vi "eventlog.vi"(7 "httpRequestID":u32) -> ()   [LabVIEW 2011]
doc: "This VI is a state machine that can be ran from a Browser."
uses:
  server/database/Users/User Record.ctl
  <vilib>/wsapi/NI_WebServices.lvlib
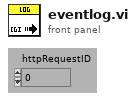
[diagram p1: front panel]
types:
  T1 = typedef "User Record.ctl" = cluster{"ixUser":i32, "sxUsername":string, "sLastName":string, "sFirstName":string, "sEmail":string, "sPassword":string, "tLoginTime":timestamp, "sLoginComputer":string, "fAdministrator":bool, "fRunSequences":bool, "fModifySequences":bool, "fRunScenarios":bool, "fModifyScenarios":bool, "fModifyTemplates":bool, "fModifyUsers":bool, "fModifyStations":bool, "fModifyFields":bool}
  T2 = typedef "Connection Refnum.ctl" = cluster{"Environment Handle":i32, "Connection Handle":i32}
  T3 = typedef "Keyed Array.ctl" = cluster{"keys":string[], "values":string[]}
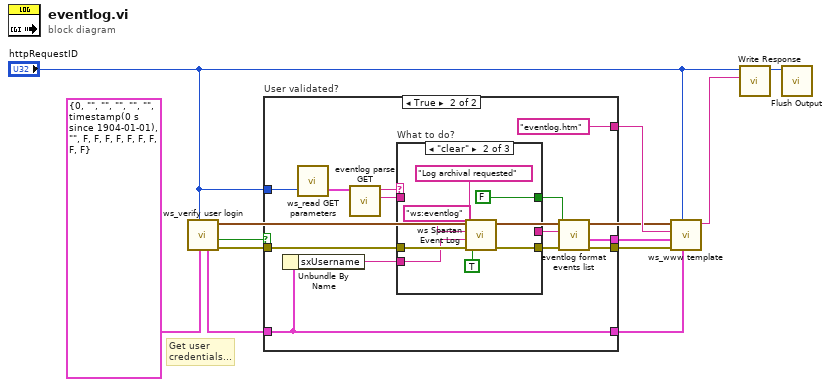
[diagram p0: block diagram]
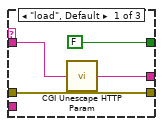
[diagram p3: hidden frame]
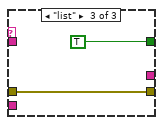
[diagram p4: hidden frame]
diagram:
  # "Get user \ncredentials..."
  n1 = call "ws_verify user login.vi"("Required Permisions"=T1 {"ixUser"=0, "sxUsername"="", "sLastName"="", "sFirstName"="", "sEmail"="", "sPassword"="", "tLoginTime"=timestamp(0 s since 1904-01-01), "sLoginComputer"="", "fAdministrator"=FALSE, "fRunSequences"=FALSE, "fModifySequences"=FALSE, "fRunScenarios"=FALSE, "fModifyScenarios"=FALSE, "fModifyTemplates"=FALSE, "fModifyUsers"=FALSE, "fModifyStations"=FALSE, "fModifyFields"=FALSE} ("User Record"), "httpRequestID"="httpRequestID") -> ("error out"=w6:errorcluster, "User Verified\nand Spartan\nAuthorized?"=w5:bool, "DB Connection Ref"=w3:T2, "User"=w4:T1)  [unwired: 6 in]
  n2 = case "User validated?" shown="True" w5 {
    tunnel: w6 -> [w14 w27]
    tunnel: [w14 w20] -> w10
    tunnel: w4 -> [w13 w19]
    tunnel: [w13 w19] -> w9
    tunnel: [_ w18] -> w11
    tunnel: [_ "eventlog.htm" ("Template (\"\")")] -> w7
    tunnel: "httpRequestID" -> [_ w15]
    frame False {
    }
    frame True {
      n3 = Unbundle By Name(w19) -> ("sxUsername"=w25:string)
      n4 = call "ws_read GET parameters.vi"("httpRequestID"=w15) -> ("GET query params"=w16:T3)  [unwired: 2 in]
      n5 = call "eventlog parse GET.vi"("GET (empty)"=w16) -> ("parameter"=w21:string, "Command"=w26:string)  [unwired: 5 out]
      n6 = case "What to do?" shown="\"clear\"" w26 {
        tunnel: w27 -> [w31 w38 w40]
        tunnel: [w31 w37 w40] -> w24
        tunnel: [FALSE FALSE TRUE] -> w23
        tunnel: w25 -> [_ w33 _]
        tunnel: [w28 _ _] -> w22
        tunnel: w21 -> [w29 _ _]
        frame "load", Default {
          n7 = call <vilib>:"CGI Unescape HTTP Param.vi"("url-encoded string"=w29) -> ("string"=w28:string)
        }
        frame "clear" {
          n8 = call "ws Spartan Event Log.vi"("Force Archive? (f)"=TRUE, "error in (no error)"=w38, "username (\"\")"=w33, "module (\"\")"="ws:eventlog", "message (\"\")"="Log archival requested") -> ("error out"=w37:errorcluster)  [unwired: 3 in]
        }
        frame "list" {
        }
      }
      n9 = call "eventlog format events list.vi"("error in (no error)"=w24, "event log (\"\": load current)"=w22, "Show Archived Logs? (f)"=w23) -> ("error out"=w20:errorcluster, "Template Keys"=w18:T3)  [unwired: 1 in, 6 out]
    }
  }
  n10 = call "ws_www template.vi"("User"=w9, "httpRequestID"="httpRequestID", "error in (no error)"=w10, "Template Keys (empty)"=w11, "Template (\"\")"=w7, "DB Connection Ref"=w3) -> ("HTTP Template Content"=w8:string)  [unwired: 5 in]
  n11 = call <vilib>:"Write Response.vi"("response string"=w8, "httpRequestID"="httpRequestID") -> ("httpRequestID out"=w12:u32)  [unwired: 8 in, 1 out]
  n12 = call <vilib>:"Flush Output.vi"("httpRequestID"=w12) -> ()  [unwired: 9 in, 2 out]
